vi "Read Value.vi"(8 "error in (no error)":errorcluster, 11 "NT Scalar in":refnum<class "NT Scalar.lvclass">) -> (0 "error out":errorcluster, 2 "value":variant, 3 "NT Scalar out":refnum<class "NT Scalar.lvclass">)   [LabVIEW 2020, in "PV Access.lvlib" / "PV Data.lvlib" / "NT Scalar.lvclass"]
uses:
  NT Scalar.lvclass
  NT Scalar.lvclass/NT Scalar.ctl
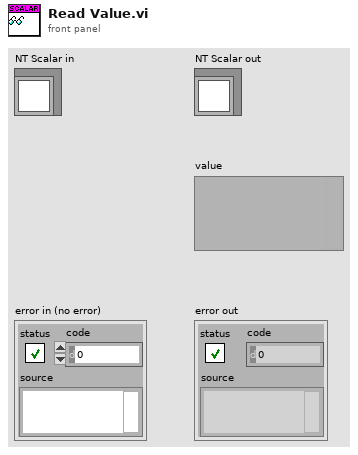
[diagram p1: front panel]
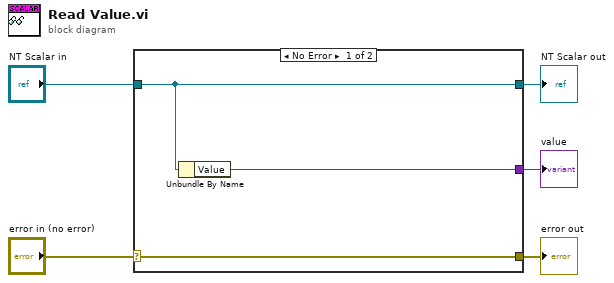
[diagram p0: block diagram]
diagram:
  n1 = case shown="No Error" "error in (no error)" {
    selector: "error in (no error)" -> [w8 w9]
    tunnel: [w8 w9] -> w4
    tunnel: [w7 w10] -> w2
    tunnel: "NT Scalar in" -> [w7 w10]
    tunnel: [w6 _] -> w1
    frame No Error {
      n2 = Unbundle By Name(w7) -> ("Value"=w6:variant)
    }
    frame Error {
    }
  }
  "error out" <- w4
  "NT Scalar out" <- w2
  "value" <- w1
